vi "LHPW Latent Heat of Evaporation of Pure Water (KJ to Kg).vi"(1 "Tceg":dbl[unit]) -> (0 "LHPW":dbl[unit])   [LabVIEW 2018]
panel:
  out "LHPW":dbl[unit](knob)
  out "Temprature of Pure Water \nKelvin Degree":dbl[unit](slide) scale=273.0..373.0
  out "Tk":dbl[unit]
  out "Temprature of Pure Water\nCentigrade Degree":dbl[unit](slide) scale=0.0..100.0
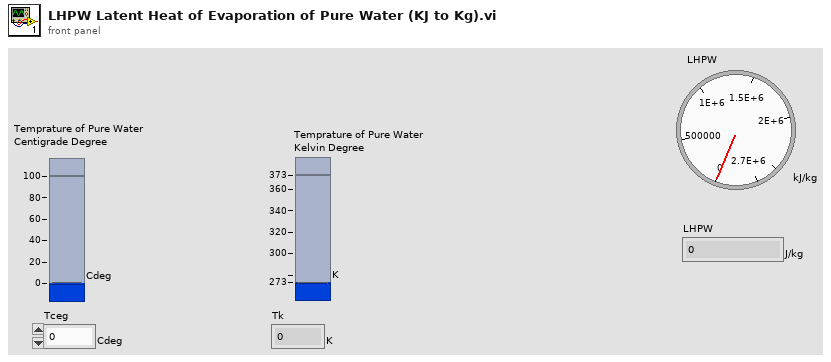
[diagram p1: front panel]
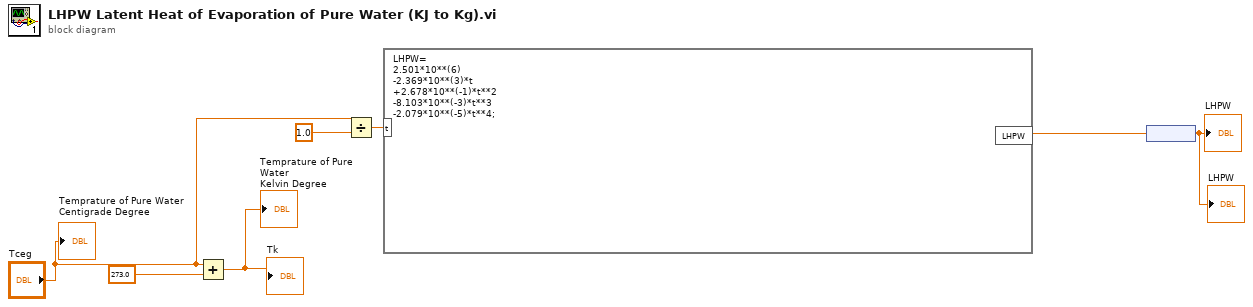
[diagram p0: block diagram]
diagram:
  n1 = Add(x="Tceg", y=dbl[unit] 273.0) -> (x+y=→"Tk" →"Temprature of Pure Water \nKelvin Degree":dbl[unit])
  n2 = Divide(x="Tceg", y=dbl[unit] 1.0) -> (x/y=w7:dbl)
  n3 = formula code="LHPW=\n2.501*10**(6)\n-2.369*10**(3)*t\n+2.678*10**(-1)*t**2\n-8.103*10**(-3)*t**3\n-2.079*10**(-5)*t**4;"("t"=w7) -> ("LHPW"=w5:dbl)
  n4 = node(w5) -> (→"LHPW" →"LHPW":dbl[unit])
  "Temprature of Pure Water\nCentigrade Degree" <- "Tceg"
